vi "Create All Message Queues.vi"(8 "error in (no error)":errorcluster[](array[cluster]), 11 "Queue Name (unnamed)":string) -> (0 "error out":errorcluster[](array[cluster]), 3 "Message Queues out":T1)   [LabVIEW 2018, in "Message Queue.lvlib"]
doc: "This VI creates and initializes all the message queues for your application. If your application requires more than one message queue, right-click the \"Message Queues\" constant above and select Open Type Def. Add the new Message Queue(s) to the type definition, then initialize them in this VI."
uses:
  Message Queue.lvlib
  All Message Queues.ctl
  Message Cluster.ctl
  Enqueue Message (Single).vi
  <userlib>/NIST/NISTErrorLib/NISTErrorLib.lvlib
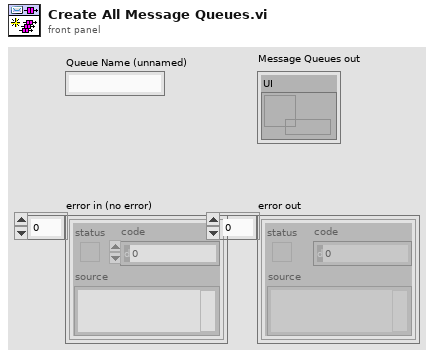
[diagram p1: front panel]
types:
  T1 = typedef "Message Queue.lvlib/All Message Queues.ctl" = cluster{"UI":refnum<queue>}
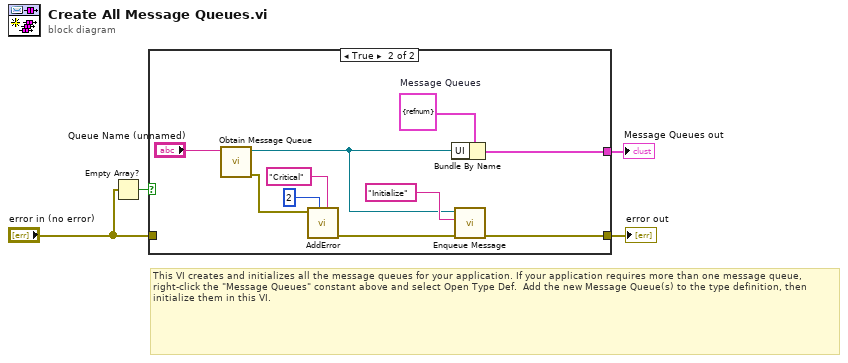
[diagram p0: block diagram]
diagram:
  # "This VI creates and initializes all the message queues for your application. If your application requires more than one message queue, right-click the \"Message Queues\" constant above and select Open Type Def.  Add the new Message Queue(s) to the type definition, then initialize them in this VI."
  n1 = Empty Array?(array="error in (no error)") -> (empty?=w1:bool)
  n2 = case shown="True" w1 {
    tunnel: [w5 w15] -> w4
    tunnel: [_ w13] -> w3
    tunnel: "error in (no error)" -> [w5 _]
    frame False {
    }
    frame True {
      w14 = T1 {"UI"=refnum}  # Message Queues
      n3 = call "Obtain Message Queue.vi"("Queue Name (unnamed)"="Queue Name (unnamed)") -> ("error out"=w9:errorcluster, "Message Queue"=w11:refnum<queue>)  [unwired: 9 in]
      n4 = call <userlib>:"AddError.vi"("Severity"="Critical", "Priority"=u8 2, "error in (no error)"=w9) -> ("ErrorArray Out"=w8:errorcluster[])  [unwired: 7 in, 1 out]
      n5 = Bundle By Name(cluster=w14, "UI"=w11) -> (w13:T1)
      n6 = call-poly "Enqueue Message.vi"("error in (no error)"=w8, "Message"="Initialize", "Message Queue"=w11) -> ("error out"=w15:errorcluster[])  [unwired: 7 in, 1 out]
    }
  }
  "Message Queues out" <- w3
  "error out" <- w4
